vi "Front Left Wheel.vi"(9 "output cluster 2":T2={"Z"=0.0, "Y"=0.0, "X"=0.0, "Rot Point X"=0.0, "Rot Point Y"=0.0, "Width / 2"=11.5, "Z Max"=16.263455967290593, "Length / 2"=11.5, "[8]"=0.0}, 10 "Pot Val in":dbl=0.880267870169171, 11 "Wheel Angle Offset":dbl=132.6) -> (0 "Drive Speed":dbl, 1 "Wheel Angle":dbl=269.7762890319989, 3 "Wheel Speed":dbl)   [LabVIEW 2019]
uses:
  <vilib>/addons/control/pid/pid.llb/PID (DBL).vi
  <vilib>/addons/control/pid/NI_PID_pid.lvlib
panel:
  in  "PID gains":T1={"proportional gain (Kc)"=0.01, "integral time (Ti, min)"=0.0, "derivative time (Td, min)"=0.0} {"derivative time (Td, min)" format="%.3f"; "integral time (Ti, min)" format="%.3f"; "proportional gain (Kc)" format="%.3f"}
  out "Requested Angle":dbl
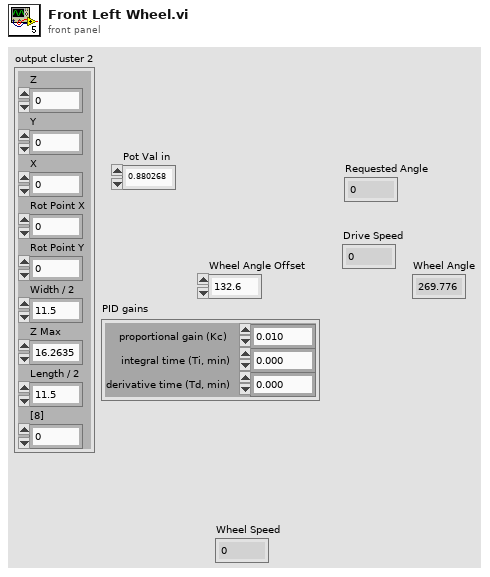
[diagram p1: front panel]
types:
  T1 = cluster{"proportional gain (Kc)":dbl, "integral time (Ti, min)":dbl, "derivative time (Td, min)":dbl}
  T2 = cluster{"Z":dbl, "Y":dbl, "X":dbl, "Rot Point X":dbl, "Rot Point Y":dbl, "Width / 2":dbl, "Z Max":dbl, "Length / 2":dbl, "[8]":dbl}
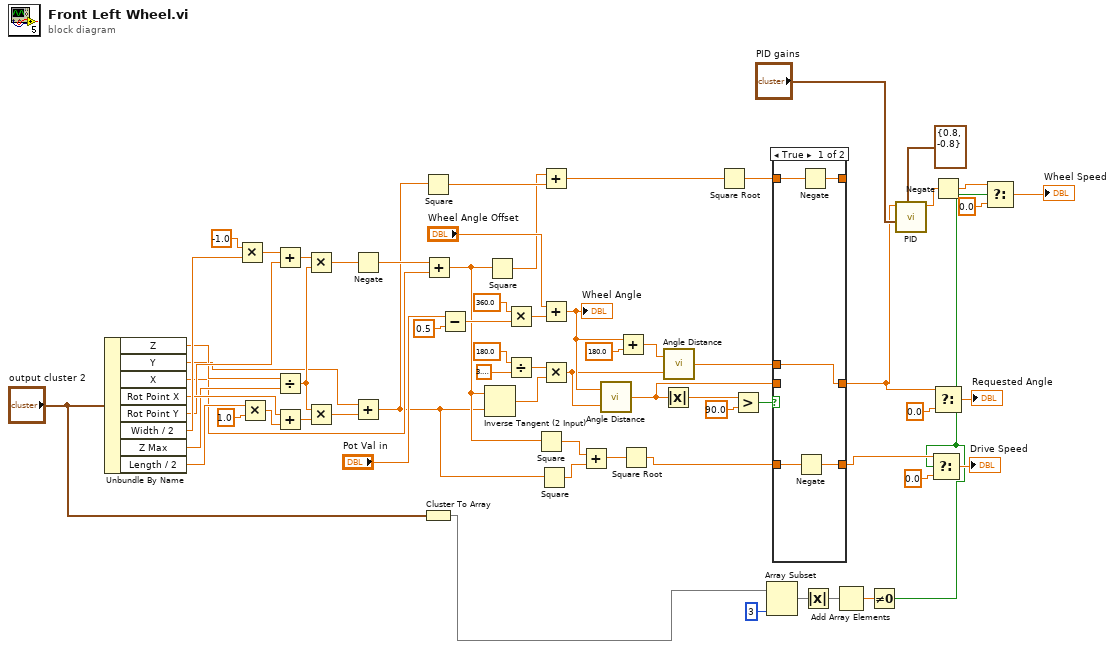
[diagram p0: block diagram]
diagram:
  n1 = Unbundle By Name("output cluster 2") -> ("Z"=w29:dbl, "Y"=w27:dbl, "X"=w26:dbl, "Rot Point X"=w31:dbl, "Rot Point Y"=w30:dbl, "Width / 2"=w63:dbl, "Z Max"=w28:dbl, "Length / 2"=w64:dbl)
  n2 = Multiply(x=-1.0, y=w63) -> (x*y=w40:dbl)
  n3 = Multiply(x=w64, y=1.0) -> (x*y=w39:dbl)
  n4 = Add(x=w40, y=w30) -> (x+y=w41:dbl)
  n5 = Divide(x=w29, y=w28) -> (x/y=w46:dbl)
  n6 = Add(x=w31, y=w39) -> (x+y=w47:dbl)
  n7 = Multiply(x=w41, y=w46) -> (x*y=w43:dbl)
  n8 = Multiply(x=w46, y=w47) -> (x*y=w44:dbl)
  n9 = Negate(x=w43) -> (-x=w42:dbl)
  n10 = Add(x=w27, y=w44) -> (x+y=w9:dbl)
  n11 = Square(x=w9) -> (x^2=w52:dbl)
  n12 = Cluster To Array(cluster="output cluster 2") -> (array=w17:dbl[])
  n13 = Add(x=w42, y=w26) -> (x+y=w10:dbl)
  n14 = Subtract(x="Pot Val in", y=0.5) -> (x-y=w61:dbl)
  n15 = Inverse Tangent (2 Input)(1:w9, 2:w10) -> (0:w53:dbl)
  n16 = Square(x=w10) -> (x^2=w45:dbl)
  n17 = Multiply(x=360.0 ("y"), y=w61) -> (x*y=w59:dbl)
  n18 = Divide(x=180.0 ("y"), y=3.141592653589793) -> (x/y=w50:dbl)
  n19 = Square(x=w10) -> (x^2=w12:dbl)
  n20 = Square(x=w9) -> (x^2=w11:dbl)
  n21 = Add(x=w45, y=w52) -> (x+y=w51:dbl)
  n22 = Add(x="Wheel Angle Offset", y=w59) -> (x+y=w54:dbl)
  "Wheel Angle" <- w54
  n23 = Multiply(x=w50, y=w53) -> (x*y=w38:dbl)
  n24 = Add(x=w12, y=w11) -> (x+y=w13:dbl)
  n25 = call "Angle Distance.vi"("target angle"=w38, "current angle"=w54) -> ("distance"=w33:dbl)
  n26 = Add(x=w54, y=180.0) -> (x+y=w55:dbl)
  n27 = Square Root(x=w13) -> (sqrt(x)=w8:dbl)
  n28 = Absolute Value(x=w33) -> (abs(x)=w36:dbl)
  n29 = call "Angle Distance.vi"("target angle"=w38, "current angle"=w55) -> ("distance"=w34:dbl)
  n30 = Square Root(x=w51) -> (sqrt(x)=w32:dbl)
  n31 = Greater?(x=w36, y=90.0) -> (0:w35:bool)
  n32 = Array Subset(array=w17, length=3) -> (w24:dbl[])  [unwired: 1 in]
  n33 = case shown="True" w35 {
    tunnel: w34 -> [w69 _]
    tunnel: w33 -> [_ w74]
    tunnel: [w70 w73] -> _
    tunnel: w32 -> [w71 w73]
    tunnel: [w69 w74] -> w3
    tunnel: [w68 w72] -> w5
    tunnel: w8 -> [w67 w72]
    frame True {
      n34 = Negate(x=w67) -> (-x=w68:dbl)
      n35 = Negate(x=w71) -> (-x=w70:dbl)
    }
    frame False {
    }
  }
  n36 = Absolute Value(x=w24) -> (abs(x)=w21:dbl[])
  n37 = Add Array Elements(numeric array=w21) -> (sum=w25:dbl)
  n38 = Not Equal To 0?(x=w25) -> (x != 0?=w4:bool)
  n39 = call-poly <vilib>:"PID.vi"("output range"=cluster{"output high":dbl, "output low":dbl} {"output high"=0.8, "output low"=-0.8}, "PID gains"="PID gains", "setpoint"=w3) -> ("output"=w1:dbl)  [unwired: 7 in, 1 out]
  n40 = Select(t=w5, s=w4, f=0.0) -> (s? t:f=→"Drive Speed":dbl)
  n41 = Negate(x=w1) -> (-x=w2:dbl)
  n42 = Select(t=w3, s=w4, f=0.0) -> (s? t:f=→"Requested Angle":dbl)
  n43 = Select(t=w2, s=w4, f=0.0) -> (s? t:f=→"Wheel Speed":dbl)
